vi "Sequence.BuildSetup.vi"(8 "error in (no error)":errorcluster, 11 "Sequence":refnum<k24>) -> (0 "error out":errorcluster, 3 "Sequence out":refnum<k24>)   [LabVIEW 2013, in "Simple Sequence Tools - Editor.lvlib"]
uses:
  Simple Sequence Tools - Editor.lvlib
  NationalInstruments.VeriStand.RealTimeSequenceDefinitionApi
  Shared/SubVIs/Constants.vi
  Shared/Simple Sequence Tools - Shared.lvlib
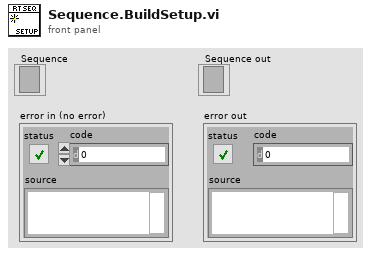
[diagram p1: front panel]
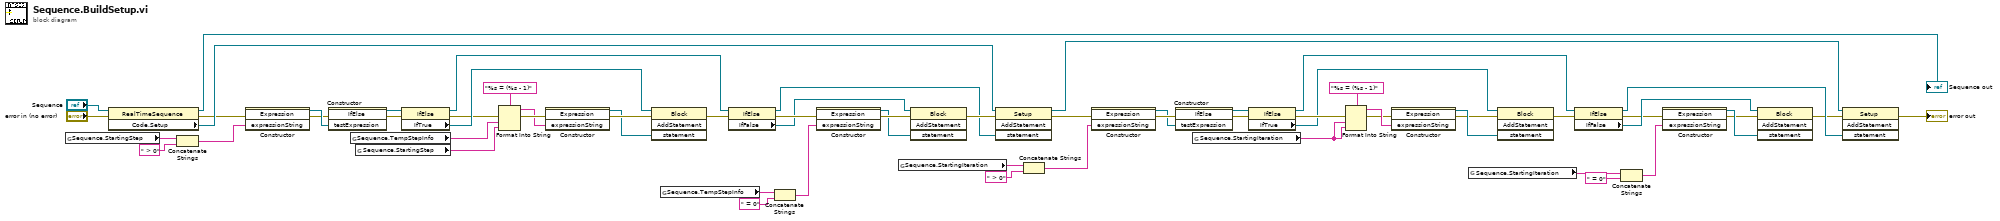
[diagram p0: block diagram]
diagram:
  n1 = global read "Constants.vi" "Sequence.StartingStep"() -> (w54:string)
  n2 = property class="RealTimeSequence"(reference="Sequence", error in="error in (no error)") -> (reference out=→"Sequence out":refnum<k24>, error out=w31:errorcluster, "Code.Setup"=w60:refnum<k24>)
  n3 = Concatenate Strings(w54, " > 0" ("string")) -> (w52:string)
  n4 = constructor class="Expression"(error in=w31, "expressionString"=w52) -> (reference out=w56:refnum<k24>, error out=w55:errorcluster)  [unwired: 2 in, 2 out]
  n5 = constructor class="IfElse"(error in=w55, "testExpression"=w56) -> (reference out=w51:refnum<k24>, error out=w49:errorcluster)  [unwired: 2 in, 2 out]
  n6 = global read "Constants.vi" "Sequence.TempStepInfo"() -> (w46:string)
  n7 = global read "Constants.vi" "Sequence.StartingStep"() -> (w45:string)
  n8 = property class="IfElse"(reference=w51, error in=w49) -> (reference out=w40:refnum<k24>, error out=w47:errorcluster, "IfTrue"=w50:refnum<k24>)
  n9 = Format Into String(format string="%s = (%s - 1)", error in=w47, w46, w45) -> (resulting string=w42:string, error out=w44:errorcluster)  [unwired: 1 in]
  n10 = constructor class="Expression"(error in=w44, "expressionString"=w42) -> (reference out=w41:refnum<k24>, error out=w43:errorcluster)  [unwired: 2 in, 2 out]
  n11 = invoke class="Block" method="AddStatement"(reference=w50, error in=w43, "statement"=w41) -> (error out=w39:errorcluster)  [unwired: 1 in, 3 out]
  n12 = global read "Constants.vi" "Sequence.TempStepInfo"() -> (w38:string)
  n13 = property class="IfElse"(reference=w40, error in=w39) -> (reference out=w29:refnum<k24>, error out=w34:errorcluster, "IfFalse"=w32:refnum<k24>)
  n14 = Concatenate Strings(w38, " = 0" ("expressionString")) -> (w35:string)
  n15 = constructor class="Expression"(error in=w34, "expressionString"=w35) -> (reference out=w33:refnum<k24>, error out=w36:errorcluster)  [unwired: 2 in, 2 out]
  n16 = global read "Constants.vi" "Sequence.StartingIteration"() -> (w4:string)
  n17 = invoke class="Block" method="AddStatement"(reference=w32, error in=w36, "statement"=w33) -> (error out=w30:errorcluster)  [unwired: 1 in, 3 out]
  n18 = invoke class="Setup" method="AddStatement"(reference=w60, error in=w30, "statement"=w29) -> (reference out=w6:refnum<k24>, error out=w9:errorcluster)  [unwired: 1 in, 2 out]
  "error out" <- w9
  n19 = Concatenate Strings(w4, " > 0" ("string")) -> (w3:string)
  n20 = constructor class="Expression"(error in=w9, "expressionString"=w3) -> (reference out=w10:refnum<k24>, error out=w11:errorcluster)  [unwired: 2 in, 2 out]
  n21 = constructor class="IfElse"(error in=w11, "testExpression"=w10) -> (reference out=w12:refnum<k24>, error out=w13:errorcluster)  [unwired: 2 in, 2 out]
  n22 = global read "Constants.vi" "Sequence.StartingIteration"() -> (w2:string)
  n23 = property class="IfElse"(reference=w12, error in=w13) -> (reference out=w7:refnum<k24>, error out=w15:errorcluster, "IfTrue"=w8:refnum<k24>)
  n24 = Format Into String(format string="%s = (%s - 1)", error in=w15, w2, w2) -> (resulting string=w18:string, error out=w16:errorcluster)  [unwired: 1 in]
  n25 = constructor class="Expression"(error in=w16, "expressionString"=w18) -> (reference out=w19:refnum<k24>, error out=w17:errorcluster)  [unwired: 2 in, 2 out]
  n26 = global read "Constants.vi" "Sequence.StartingIteration"() -> (w1:string)
  n27 = invoke class="Block" method="AddStatement"(reference=w8, error in=w17, "statement"=w19) -> (error out=w20:errorcluster)  [unwired: 1 in, 3 out]
  n28 = property class="IfElse"(reference=w7, error in=w20) -> (reference out=w28:refnum<k24>, error out=w24:errorcluster, "IfFalse"=w26:refnum<k24>)
  n29 = Concatenate Strings(w1, " = 0" ("expressionString")) -> (w23:string)
  n30 = constructor class="Expression"(error in=w24, "expressionString"=w23) -> (reference out=w25:refnum<k24>, error out=w22:errorcluster)  [unwired: 2 in, 2 out]
  n31 = invoke class="Block" method="AddStatement"(reference=w26, error in=w22, "statement"=w25) -> (error out=w27:errorcluster)  [unwired: 1 in, 3 out]
  n32 = invoke class="Setup" method="AddStatement"(reference=w6, error in=w27, "statement"=w28) -> ()  [unwired: 1 in, 4 out]
